vi "Configuration 2.0 JSON Unflatten.vi"(8 "error in (no error)":errorcluster, 11 "dsf configuration json":string) -> (0 "error out":errorcluster, 3 "configuration 2.0":T1={"custom settings"=[], "plugins"=[{"core settings"={"component"="", "values"=[]}, "component settings"=[], "threads"=[{"core settings"={"component"="", "values"=[]}, "component settings"=[], "transfer groups"=[{"core settings"={"component"="Group", "values"=[]}, "component settings"=[], "transfers"=[{"core settings"={"component"="Transfer", "values"=[]}, "component settings"=[], "channels"=[{"core settings"={"component"="Channel", "values"=[]}, "component settings"=[]}]}]}]}]}]})   [LabVIEW 2020, in "DSF Core.lvlib" / "Configuration Session.lvclass"]
uses:
  Configuration Session.lvclass
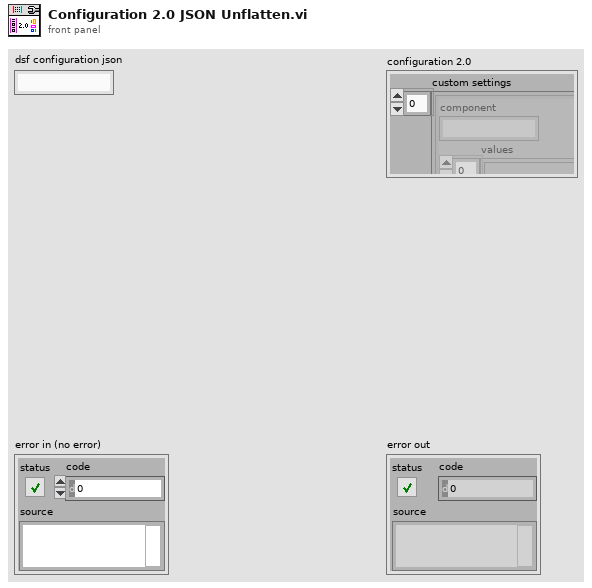
[diagram p1: front panel]
types:
  T1 = cluster{"custom settings":cluster{"component":string, "values":cluster{"key":string, "value":string}[]}[], "plugins":cluster{"core settings":cluster{"component":string, "values":cluster{"key":string, "value":string}[]}, "component settings":cluster{"component":string, "values":cluster{"key":string, "value":string}[]}[], "threads":cluster{"core settings":cluster{"component":string, "values":cluster{"key":string, "value":string}[]}, "component settings":cluster{"component":string, "values":cluster{"key":string, "value":string}[]}[], "transfer groups":cluster{"core settings":cluster{"component":string, "values":cluster{"key":string, "value":string}[]}, "component settings":cluster{"component":string, "values":cluster{"key":string, "value":string}[]}[], "transfers":cluster{"core settings":cluster{"component":string, "values":cluster{"key":string, "value":string}[]}, "component settings":cluster{"component":string, "values":cluster{"key":string, "value":string}[]}[], "channels":cluster{"core settings":cluster{"component":string, "values":cluster{"key":string, "value":string}[]}, "component settings":cluster{"component":string, "values":cluster{"key":string, "value":string}[]}[]}[]}[]}[]}[]}[]}
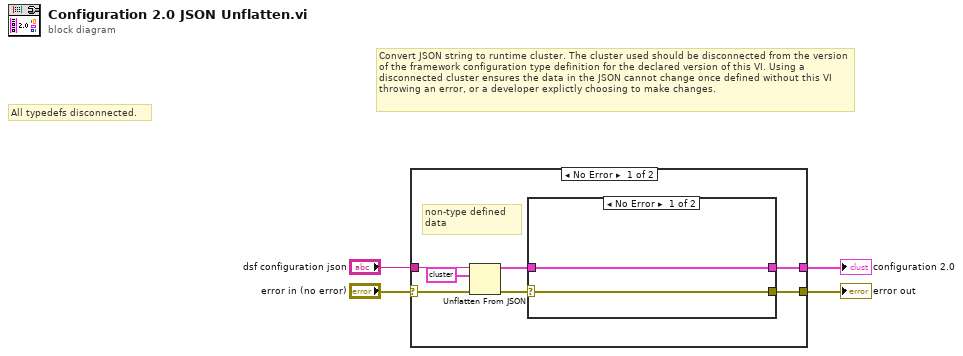
[diagram p0: block diagram]
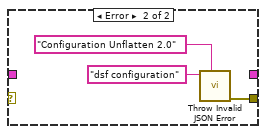
[diagram p2: hidden frame]
diagram:
  # "All typedefs disconnected."
  # "Convert JSON string to runtime cluster. The cluster used should be disconnected from the version of the framework configuration type definition for the declared version of this VI. Using a disconnected cluster ensures the data in the JSON cannot change once defined without this VI throwing an error, or a developer explictly choosing to make changes."
  n1 = case shown="No Error" "error in (no error)" {
    selector: "error in (no error)" -> [w6 w17]
    tunnel: "dsf configuration json" -> [w11 _]
    tunnel: [w9 w17] -> w3
    tunnel: [w7 _] -> w1
    frame No Error {
      # "non-type defined data"
      n2 = Unflatten From JSON(JSON string=w11, type and defaults=T1 {"custom settings"=[], "plugins"=[{"core settings"={"component"="", "values"=[]}, "component settings"=[], "threads"=[{"core settings"={"component"="", "values"=[]}, "component settings"=[], "transfer groups"=[{"core settings"={"component"="Group", "values"=[]}, "component settings"=[], "transfers"=[{"core settings"={"component"="Transfer", "values"=[]}, "component settings"=[], "channels"=[{"core settings"={"component"="Channel", "values"=[]}, "component settings"=[]}]}]}]}]}]} ("configuration 2.0"), error in (no error)=w6) -> (value=w8:T1, error out=w10:errorcluster)  [unwired: 4 in]
      n3 = case shown="No Error" w10 {
        selector: w10 -> [w13 _]
        tunnel: [w13 w16] -> w9
        tunnel: w8 -> [w12 _]
        tunnel: [w12 _] -> w7
        frame No Error {
        }
        frame Error {
          n4 = call "Throw Invalid JSON Error.vi"("error source vi name"="Configuration Unflatten 2.0", "name"="dsf configuration") -> ("error out"=w16:errorcluster)  [unwired: 9 in]
        }
      }
    }
    frame Error {
    }
  }
  "error out" <- w3
  "configuration 2.0" <- w1
